vi "Read Relay Test State.vi"(8 "error in (no error)":errorcluster, 11 "VGC in":refnum<class "PL Inficon VGC.lvclass">) -> (0 "error out":errorcluster, 1 "relays":T1, 2 "state":u16(ring) items=["off", "on"], 3 "VGC out":refnum<class "PL Inficon VGC.lvclass">)   [LabVIEW 2015, in "PL Inficon VGC.lvclass"]
doc: "Reads relay test state."
uses:
  PL Inficon VGC.lvclass
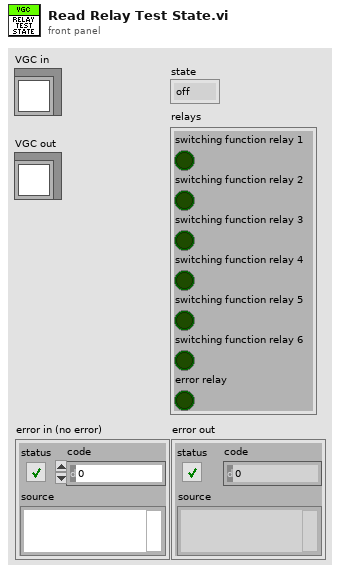
[diagram p1: front panel]
types:
  T1 = cluster{"switching function relay 1":bool, "switching function relay 2":bool, "switching function relay 3":bool, "switching function relay 4":bool, "switching function relay 5":bool, "switching function relay 6":bool, "error relay":bool}
  T2 = cluster{"Boolean array[0]":bool, "Boolean array[1]":bool, "Boolean array[2]":bool, "Boolean array[3]":bool, "Boolean array[4]":bool, "Boolean array[5]":bool, "Boolean array[6]":bool}
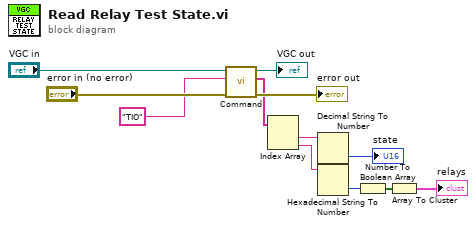
[diagram p0: block diagram]
diagram:
  n1 = call "Command.vi"("error in (no error)"="error in (no error)", "command"="TIO", "VGC in"="VGC in") -> ("error out"=→"error out":errorcluster, "response data"=w3:string[], "VGC out"=→"VGC out":refnum<class "PL Inficon VGC.lvclass">)  [unwired: 6 in]
  n2 = Index Array(array=w3) -> (element #1=w6:string, element #2=w5:string)  [unwired: 2 in]
  n3 = Decimal String To Number(string=w6) -> (number=→"state":i32)  [unwired: 2 in, 1 out]
  n4 = Hexadecimal String To Number(string=w5) -> (number=w4:u32)  [unwired: 2 in, 1 out]
  n5 = Number To Boolean Array(number=w4) -> (Boolean array=w7:bool[])
  n6 = Array To Cluster(array=w7) -> (cluster=→"relays":T2)
